vi "Get or Set Recording Directory and Duration.vi"(5 "mode":enum16{"Get", "Set"}(ring), 6 "error in (no error)":errorcluster, 7 "log duration in":dbl, 8 "log directory in":path, 9 "Message Data":variant) -> (0 "error out":errorcluster, 1 "log duration out":dbl, 2 "log directory out":path, 3 "Variant":variant)   [LabVIEW 2024, in "DSA_CFG_ACQ.lvlib"]
uses:
  DSA_CFG_ACQ.lvlib
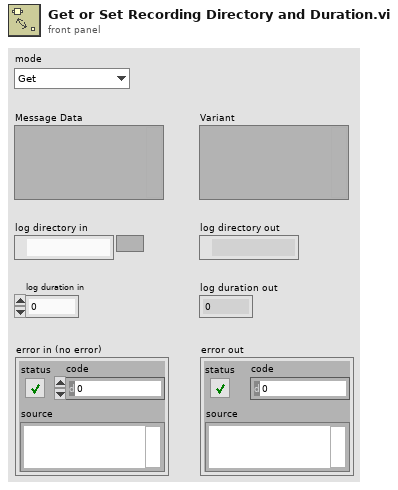
[diagram p1: front panel]
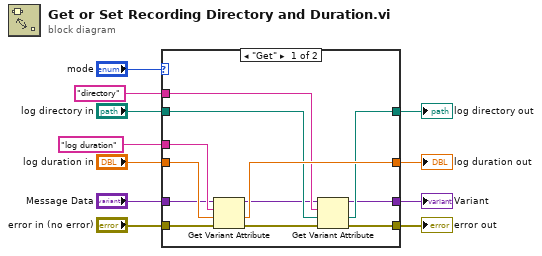
[diagram p0: block diagram]
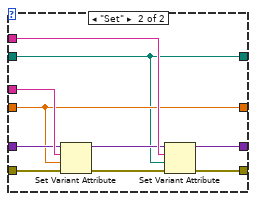
[diagram p2: hidden frame]
diagram:
  n1 = case shown="\"Get\"" "mode" {
    tunnel: "error in (no error)" -> [w23 w33]
    tunnel: [w22 w25] -> w10
    tunnel: [w21 w24] -> w9
    tunnel: "log duration in" -> [w20 w25]
    tunnel: "log directory in" -> [w19 w24]
    tunnel: "directory" ("name") -> [w18 w32]
    tunnel: "log duration" ("name") -> [w17 w31]
    tunnel: [w16 w30] -> w4
    tunnel: "Message Data" -> [w15 w29]
    tunnel: [w14 w28] -> w2
    frame "Get" {
      n2 = Get Variant Attribute(Variant=w15, name=w17, default value (empty Variant)=w20, error in=w23) -> (duplicate Variant=w12:variant, value=w22:dbl, error out=w13:errorcluster)  [unwired: 1 out]
      n3 = Get Variant Attribute(Variant=w12, name=w18, default value (empty Variant)=w19, error in=w13) -> (duplicate Variant=w16:variant, value=w21:path, error out=w14:errorcluster)  [unwired: 1 out]
    }
    frame "Set" {
      n4 = Set Variant Attribute(Variant=w29, name=w31, value=w25, error in=w33) -> (Variant out=w26:variant, error out=w27:errorcluster)  [unwired: 1 out]
      n5 = Set Variant Attribute(Variant=w26, name=w32, value=w24, error in=w27) -> (Variant out=w30:variant, error out=w28:errorcluster)  [unwired: 1 out]
    }
  }
  "log duration out" <- w10
  "log directory out" <- w9
  "Variant" <- w4
  "error out" <- w2
